vi "HatchRectIsland.vi"(10 "HatchPow":T6, 11 "RectHatch":T5={"Width"=1.0, "Height"=2.0, "Angle"=45.0, "OffX"=0.1, "OffY"=0.1, "Spacing"=0.1, "IslandSize"=0.1} {"IslandSize" format="%#_13g"; "Spacing" format="%#_13g"; "OffY" format="%#_13g"; "OffX" format="%#_13g"; "Height" format="%#_13g"; "Width" format="%#_13g"}) -> (3 "PathSupreme":T1)   [LabVIEW 2014]
uses:
  TypeDefs/PowerSpeed.ctl
  TypeDefs/RectHatch.ctl
  TypeDefs/PathSupreme.ctl
  PSup2SCAN/Sub/VelocityProfile.ctl
  PSup2SCAN/Sub/PathCut.ctl
  PSup2SCAN/Sub/Segment.ctl
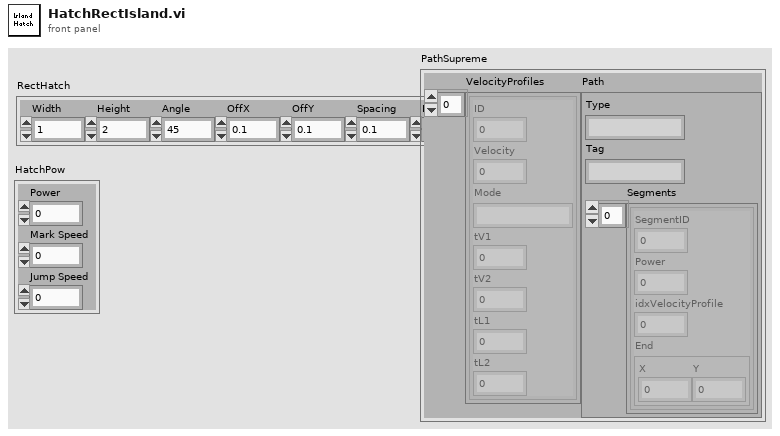
[diagram p1: front panel]
types:
  T1 = typedef "PathSupreme.ctl" = cluster{"VelocityProfiles":T2[], "Path":T3}
  T2 = typedef "VelocityProfile.ctl" = cluster{"ID":u32, "Velocity":dbl, "Mode":string, "tV1":u32, "tV2":u32, "tL1":u32, "tL2":u32}
  T3 = typedef "PathCut.ctl" = cluster{"Type":string, "Tag":string, "Segments":T4[]}
  T4 = typedef "Segment.ctl" = cluster{"SegmentID":u16, "Power":sgl, "idxVelocityProfile":u16, "End":cluster{"X":sgl, "Y":sgl}}
  T5 = typedef "RectHatch.ctl" = cluster{"Width":dbl, "Height":dbl, "Angle":sgl, "OffX":dbl, "OffY":dbl, "Spacing":dbl, "IslandSize":dbl}
  T6 = typedef "PowerSpeed.ctl" = cluster{"Power":dbl, "Mark Speed":dbl, "Jump Speed":dbl}
  T7 = typedef "Point2DwSlope.ctl" = cluster{"X":sgl, "Y":sgl, "Slope":dbl}
  T8 = cluster{"Xmin":dbl, "Xmax":dbl, "Ymin":dbl, "Ymax":dbl}
  T9 = typedef "Poly2DwSlope.ctl" = cluster{"VertexArray":T7[]}
  T10 = cluster{"VertexArray":T7[], "OnOffAr":enum16{"On", "Off"}[]}
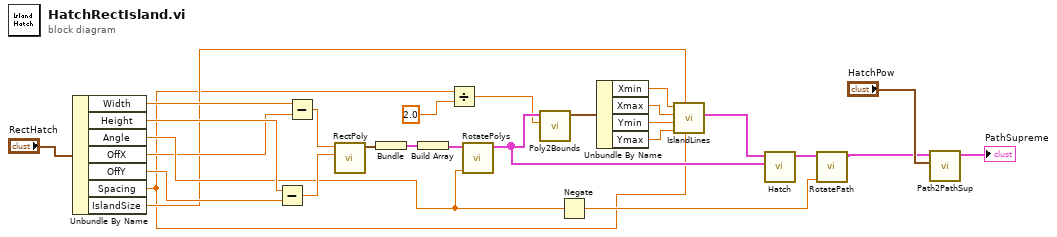
[diagram p0: block diagram]
diagram:
  n1 = Unbundle By Name("RectHatch") -> ("Width"=w11:dbl, "Height"=w10:dbl, "Angle"=w9:sgl, "OffX"=w8:dbl, "OffY"=w7:dbl, "Spacing"=w2:dbl, "IslandSize"=w3:dbl)
  n2 = Subtract(x=w10, y=w7) -> (x-y=w15:dbl)
  n3 = Subtract(x=w11, y=w8) -> (x-y=w16:dbl)
  n4 = call "RectPoly.vi"("Height"=w15, "Width"=w16) -> ("VertexArray"=w27:T7[])  [unwired: 9 in]
  n5 = Bundle("VertexArray"=w27) -> (w26:cluster{"VertexArray":T7[]})  [unwired: 1 in]
  n6 = Build Array(w26) -> (w20:cluster{"VertexArray":T7[]}[])
  n7 = Divide(x=w2, y=2.0) -> (x/y=w4:dbl)
  n8 = call "RotatePolys.vi"("Angle"=w9, "Polys"=w20) -> ("RotatedPolys"=w19:cluster{cluster{sgl, sgl, "Slope":dbl}[]}[])  [unwired: 9 in]
  n9 = call "Poly2Bounds.vi"("Border"=w4, "Polys"=w19) -> ("Bounds"=w6:T8)  [unwired: 9 in]
  n10 = Negate(x=w9) -> (-x=w17:sgl)
  n11 = Unbundle By Name(w6) -> ("Xmin"=w25:dbl, "Xmax"=w24:dbl, "Ymin"=w23:dbl, "Ymax"=w22:dbl)
  n12 = call "IslandLines.vi"("Spacing"=w2, "IslandSize"=w3, "yMax"=w22, "yMin"=w23, "xMax"=w24, "xMin"=w25) -> ("Poly2D"=w21:T9)  [unwired: 4 in, 1 out]
  n13 = call "Hatch.vi"("Polys"=w19, "Hatch"=w21) -> ("Path"=w18:T10)  [unwired: 9 in]
  n14 = call "RotatePath.vi"("Angle"=w17, "Path"=w18) -> ("RotatedPath"=w1:T10)  [unwired: 9 in]
  n15 = call "Path2PathSup.vi"("PowerSpeed"="HatchPow", "Combined"=w1) -> ("PathSupreme"=→"PathSupreme":T1)  [unwired: 9 in]
